vi "Set_Meas_Mode.vi"(0 "VISA in":refnum<visa-resource-name>, 1 "Measurement mode":enum16{"MODE 1", "MODE 2"}(ring), 2 "error in (no error)":errorcluster) -> (3 "VISA out":refnum<visa-resource-name>, 6 "error out":errorcluster)   [LabVIEW 2017, in "GP22_TDC_Arduinoed.lvlib"]
doc: "Set's the measurement mode of the GP22. \n\nFrom the datasheet, MODE 1 ranges from 3.5ns to 2.4us, whereas MODE 2 goes from 700ns to 4ms"
uses:
  GP22_TDC_Arduinoed.lvlib
  <vilib>/regexp/Match Regular Expression.xnode
panel:
  out "read buffer":string
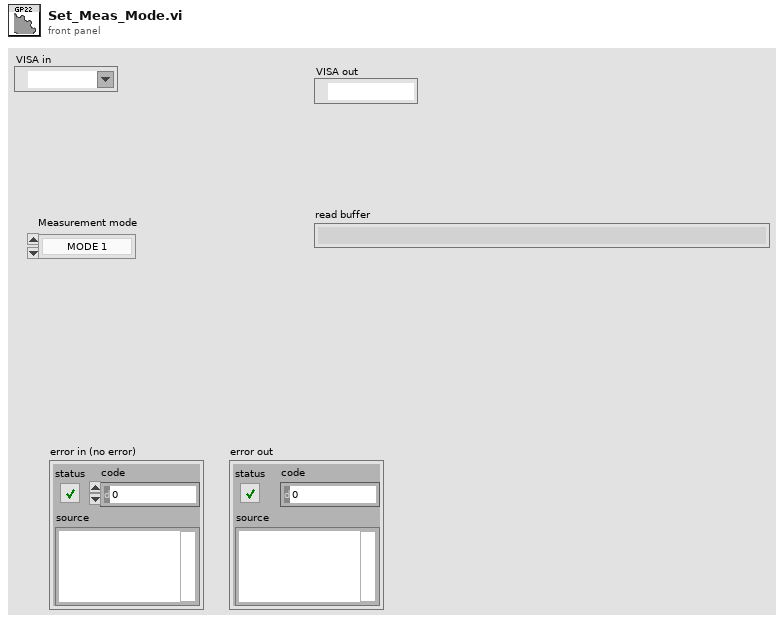
[diagram p1: front panel]
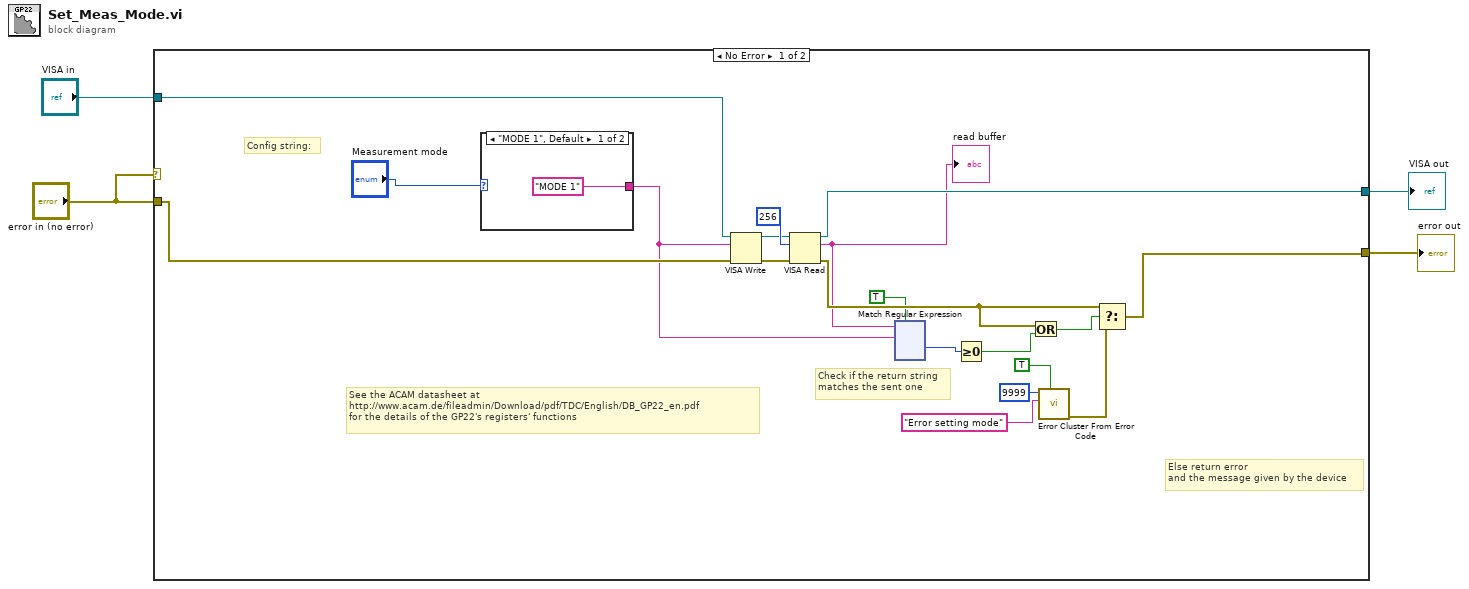
[diagram p0: block diagram]
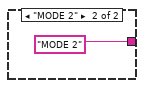
[diagram p2: hidden frame]
diagram:
  n1 = case shown="No Error" "error in (no error)" {
    tunnel: [w23 w141] -> w4
    tunnel: "error in (no error)" -> [w14 w141]
    tunnel: [w17 w140] -> w2
    tunnel: "VISA in" -> [w16 w140]
    frame No Error {
      # "See the ACAM datasheet at \nhttp://www.acam.de/fileadmin/Download/pdf/TDC/English/DB_GP22_en.pdf\nfor the details of the GP22's registers' functions"
      # "Config string:"
      # "Else return error\nand the message given by the device"
      # "Check if the return string\nmatches the sent one"
      n2 = case shown="\"MODE 1\", Default" "Measurement mode" {
        tunnel: ["MODE 1" "MODE 2"] -> w12
        frame "MODE 1", Default {
        }
        frame "MODE 2" {
        }
      }
      n3 = VISA Write(VISA resource name=w16, write buffer=w12, error in (no error)=w14) -> (VISA resource name out=w20:refnum<visa-resource-name>, error out=w21:errorcluster)  [unwired: 1 out]
      n4 = VISA Read(VISA resource name=w20, byte count=u32 256, error in (no error)=w21) -> (VISA resource name out=w17:refnum<visa-resource-name>, read buffer=w5:string, error out=w19:errorcluster)  [unwired: 1 out]
      "read buffer" <- w5
      n5 = xnode "Match Regular Expression"("input string"=w5, "regular expression"=w12, "ignore case? (F)"=TRUE) -> ("offset past match"=w11:i32)  [unwired: 3 in, 4 out]
      n6 = Greater Or Equal To 0?(x=w11) -> (x >= 0?=w6:bool)
      n7 = Or(x=w19, y=w6) -> (x .or. y?=w18:bool)
      n8 = call <vilib>:"Error Cluster From Error Code.vi"("show call chain? (False)"=TRUE, "error message (\"\")"="Error setting mode" ("string"), "error code (0)"=9999) -> ("error out"=w7:errorcluster)  [unwired: 6 in]
      n9 = Select(t=w19, s=w18, f=w7) -> (s? t:f=w23:errorcluster)
    }
    frame Error {
    }
  }
  "error out" <- w4
  "VISA out" <- w2
